vi "Strip Class Function Name.vi"(4 "Strip vi extension(T)":bool=TRUE, 5 "File Full Path Name":string="NEVSTOP-MemBuffer.lvlib:memBuffer.lvclass:replace memory subs") -> (0 "library name":string, 1 "Class name":string, 2 "Function Name":string="replace memory subs")   [LabVIEW 2017]
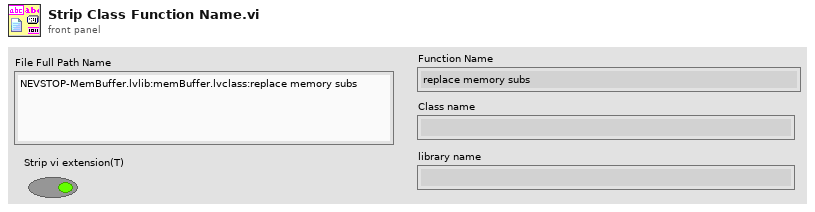
[diagram p1: front panel]
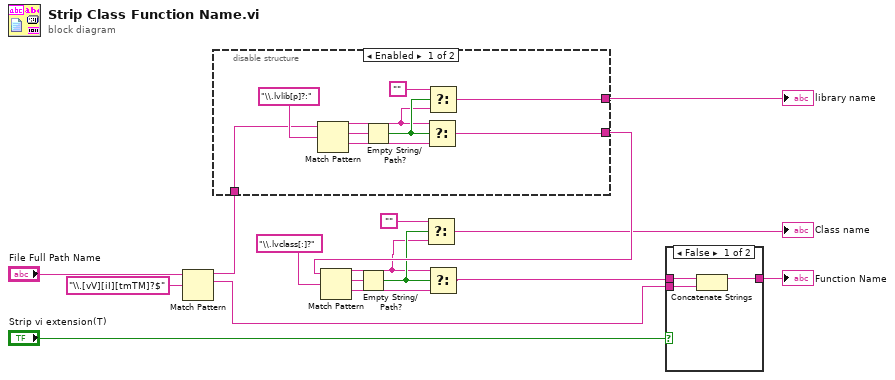
[diagram p0: block diagram]
diagram:
  n1 = Match Pattern(string="File Full Path Name", regular expression="\\.[vV][iI][tmTM]?$") -> (before substring=w8:string, match substring=w10:string)  [unwired: 1 in, 2 out]
  n2 = disable-structure shown="Enabled" {
    disable-tunnel: w8 -> [w22 w26]
    disable-tunnel: [w21 w26] -> w7
    disable-tunnel: [w19 _] -> w5
    frame Enabled {
      n3 = Match Pattern(string=w22, regular expression="\\.lvlib[p]?:") -> (before substring=w18:string, match substring=w24:string, after substring=w23:string)  [unwired: 1 in, 1 out]
      n4 = Empty String/Path?(string/path=w24) -> (empty?=w20:bool)
      n5 = Select(t=w18, s=w20, f=w23) -> (s? t:f=w21:string)
      n6 = Select(t="", s=w20, f=w18) -> (s? t:f=w19:string)
    }
    frame Disabled {
    }
  }
  "library name" <- w5
  n7 = Match Pattern(string=w7, regular expression="\\.lvclass[:]?") -> (before substring=w2:string, match substring=w14:string, after substring=w15:string)  [unwired: 1 in, 1 out]
  n8 = Empty String/Path?(string/path=w14) -> (empty?=w4:bool)
  n9 = Select(t="", s=w4, f=w2) -> (s? t:f=→"Class name":string)
  n10 = Select(t=w2, s=w4, f=w15) -> (s? t:f=w6:string)
  n11 = case shown="False" "Strip vi extension(T)" {
    tunnel: w6 -> [w29 w30]
    tunnel: [w28 w30] -> w11
    tunnel: w10 -> [w27 _]
    frame False {
      n12 = Concatenate Strings(w29, w27) -> (w28:string)
    }
    frame True {
    }
  }
  "Function Name" <- w11
